vi "Delta Linear movement after Calibration.vi"() -> ()   [LabVIEW 2019]
panel:
  in  "z0":dbl(slide) scale=-135.0..50.0
  in  "y0":dbl(slide) scale=-115.0..115.0
  in  "x0":dbl(slide) scale=-115.0..115.0
  in  "RealWorldXY":cluster{"X":dbl, "Y":dbl}[][](array[cluster])=[[{"X"=-87.41918672815254, "Y"=-97.69950478545138}, {"X"=-44.676485154645185, "Y"=-97.86512942901233}, {"X"=1.0693055499785054, "Y"=-96.7577952889925}, {"X"=46.64075452454025, "Y"=-96.29119342235651}, {"X"=92.22082906177734, "Y"=-94.31936241201021}], [{"X"=-87.32274234871466, "Y"=-53.379030153432595}, {"X"=-43.46989684226859, "Y"=-51.8943192724522}, {"X"=0.9696666097077349, "Y"=-50.19260805869147}, {"X"=46.92217377535491, "Y"=-48.82417436459591}, {"X"=92.86040893315193, "Y"=-47.29622999450278}], [{"X"=-88.21280481186528, "Y"=-8.543006319347361}, {"X"=-42.795865235008016, "Y"=-7.3111011709588976}, {"X"=1.5816838876191233, "Y"=-6.615970435553383}, {"X"=47.03370209011219, "Y"=-4.021048175235278}, {"X"=93.9643907170363, "Y"=-1.4217991071066687}], [{"X"=-90.43482001089998, "Y"=35.789019295879484}, {"X"=-43.4846477445188, "Y"=38.11224916526762}, {"X"=2.3229241868558685, "Y"=39.03811614961179}, {"X"=46.863686527489115, "Y"=42.268175048978364}, {"X"=96.00471066315937, "Y"=43.92236372382627}], [{"X"=-93.42540075638188, "Y"=79.55955711607037}, {"X"=-44.09351543445324, "Y"=80.92850550222232}, {"X"=2.026996037323034, "Y"=84.04279899262731}, {"X"=49.043392430832846, "Y"=85.91841796569378}, {"X"=98.98878177149534, "Y"=89.88724663362977}]]
  in  "DeltaXY":cluster{dbl, dbl}[][](array[cluster])=[[{-100.0, -100.0}, {-50.0, -100.0}, {0.0, -100.0}, {50.0, -100.0}, {100.0, -100.0}], [{-100.0, -50.0}, {-50.0, -50.0}, {0.0, -50.0}, {50.0, -50.0}, {100.0, -50.0}], [{-100.0, 0.0}, {-50.0, 0.0}, {0.0, 0.0}, {50.0, 0.0}, {100.0, 0.0}], [{-100.0, 50.0}, {-50.0, 50.0}, {0.0, 50.0}, {50.0, 50.0}, {100.0, 50.0}], [{-100.0, 100.0}, {-50.0, 100.0}, {0.0, 100.0}, {50.0, 100.0}, {100.0, 100.0}]]
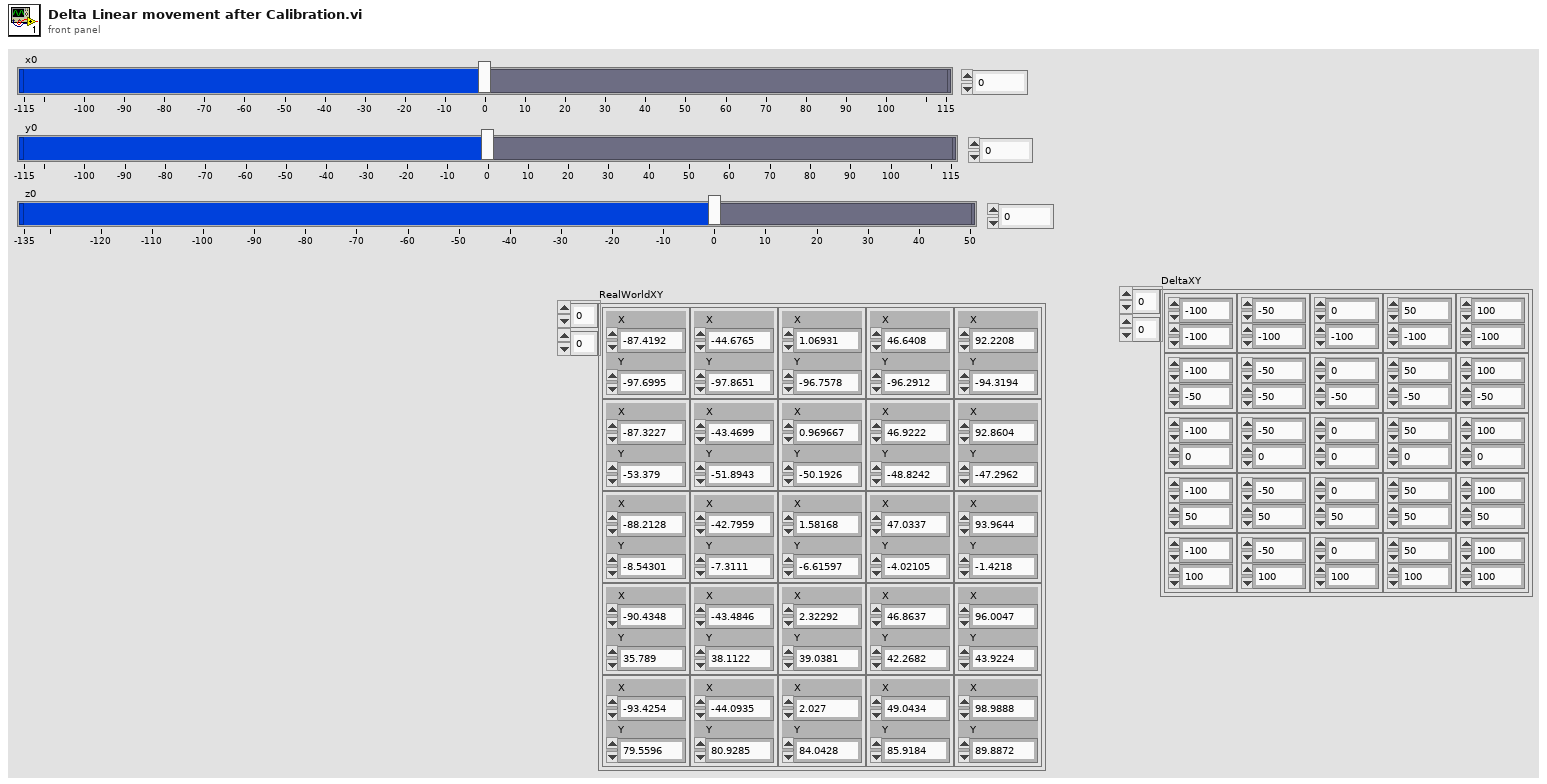
[diagram p1: front panel]
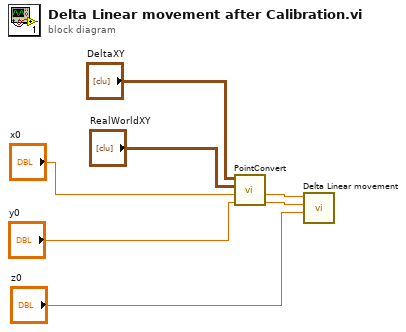
[diagram p0: block diagram]
diagram:
  n1 = call "PointConvert.vi"("RealWorldY"="y0", "RealWorldX"="x0", "RealWorldXY"="RealWorldXY", "DeltaXY"="DeltaXY") -> ("DeltaY"=w3:dbl, "DeltaX"=w4:dbl)  [unwired: 5 in, 1 out]
  n2 = call "Delta Linear movement.vi"("z0"="z0", "y0"=w3, "x0"=w4) -> ()  [unwired: 8 in, 1 out]
